vi "Example_OE1201 Control.vi"() -> ()   [LabVIEW 2011]
panel:
  in  "Sample count":u32
  out "Gain Overlaod":bool
  in  "Remote Mode":u16(ring) items=["USB", "RS232"]
  out "Freq":dbl
  out "xita":dbl
  out "R":dbl
  out "Input Overlaod":bool
  out "PLL Lock":bool
  out "Error":string
  out "Serial Versions":string
  in  "Table":T1(tab) caption="选项卡控件"
  in  "OE1201_Configure Input Filter":T2 {"Input Notch Filter" items=["None", "50Hz", "100Hz", "Both"]; "Input Coupling" items=["AC", "DC"]; "Input Shield Grounding" items=["Float", "Ground"]; "Input Source" items=["A", "B", "I-1M", "I-100M"]}
  in  "OE1201_Configure Ref Phase":T3={"Internal Frequency(Hz)"=1000.0, "External Ref Trigger"=0, "Reference Source"=0, "Phase  (degree)"=0.0} {"Phase  (degree)" format="%#.2g"; "Reference Source" items=["External", "Internal"]; "External Ref Trigger" items=["TTL Rising Edge", "Sine Zero Crossing"]; "Internal Frequency(Hz)" min=0.001 max=120000.0 format="%#_10g"}
  in  "OE1201_Configure Sens and Filter":T4={"Dynamic Reserve"=1, "Sensitivity "=24, "Time Constant "=9, "Low Pass Filter Slope "=1, "Enable Sync Filter "=0} {"Enable Sync Filter" items=["OFF", "ON"]; "Low Pass Filter Slope" items=["6 dB/oct", "12 dB/oct", "18 db/oct", "24 dB/oct"]; "Time Constant" items=["10 us", "30 us", "100 us", "300 us", "1 ms", "3 ms", "10 ms", "30 ms", "100 ms", "300 ms", "1 s", "3 s", "10 s", "30 s", "100 s", "300 s", "1 ks", "3 ks"]; "Sensitivity" items=["2 nV/fA", "5 nV/fA", "10 nV/fA", "20 nV/fA", "50 nV/fA", "100 nV/fA", "200 nV/fA", "500 nV/fA", "1 uV/pA", "2 uV/pA", "5 uV/pA", "10 uV/pA", "20 uV/pA", "50 uV/pA", "100 uV/pA", "200 uV/pA", "500 uV/pA", "1 mV/nA", "2 mV/nA", "5 mV/nA", "10 mV/nA", "20 mV/nA", "50 mV/nA", "100 mV/nA", "200 mV/nA", "500 mV/nA", "1 V/uA"]; "Dynamic Reserve" items=["High Reserve", "Normal", "Low Noise"]}
  in  "OE1201_Configure Channel Out":T5={"CH 1"=0, "CH 2"=0, "CH2 Offset(%)"=0.0, "CH1 Offset(%)"=0.0, "CH2 Expand"=1, "CH1 Expand"=1} {"CH1 Expand" min=1 max=256; "CH2 Expand" min=1 max=256; "CH1 Offset(%)" min=-100.0 max=100.0 format="%#.2g"; "CH2 Offset(%)" min=-100.0 max=100.0 format="%#.2g"; "CH 2" items=["R"=3, "X"=1, "Y"=2, "θ"=4]; "CH 1" items=["R"=3, "X"=1, "Y"=2, "θ"=4]}
  in  "OE1201_Configure Sine Out":cluster{"Sine Output Amplitude (V)":dbl}={"Sine Output Amplitude (V)"=0.1} {"Sine Output Amplitude (V)" min=0.1 max=1.0 format="%.3f"}
  in  "OE1201_Configure Harmonic":cluster{"Harmonic":u16}={"Harmonic"=1} {"Harmonic" min=1 max=32767}
  in  "Sample Rate":dbl=0.1 min=0.1 max=100.0
  in  "Save Button":bool
  in  "file path":path
  out "Status":string
  in  "Connect":bool
  in  "VISA resource name":refnum<visa-resource-name>
  in  "Baud Rate (921600)":u32=921600
  # "Tel          :   +86-020-84133345\nWebsite  :   www.ssi-instrument.com\nE-mail     :   support@si-instrument.com"
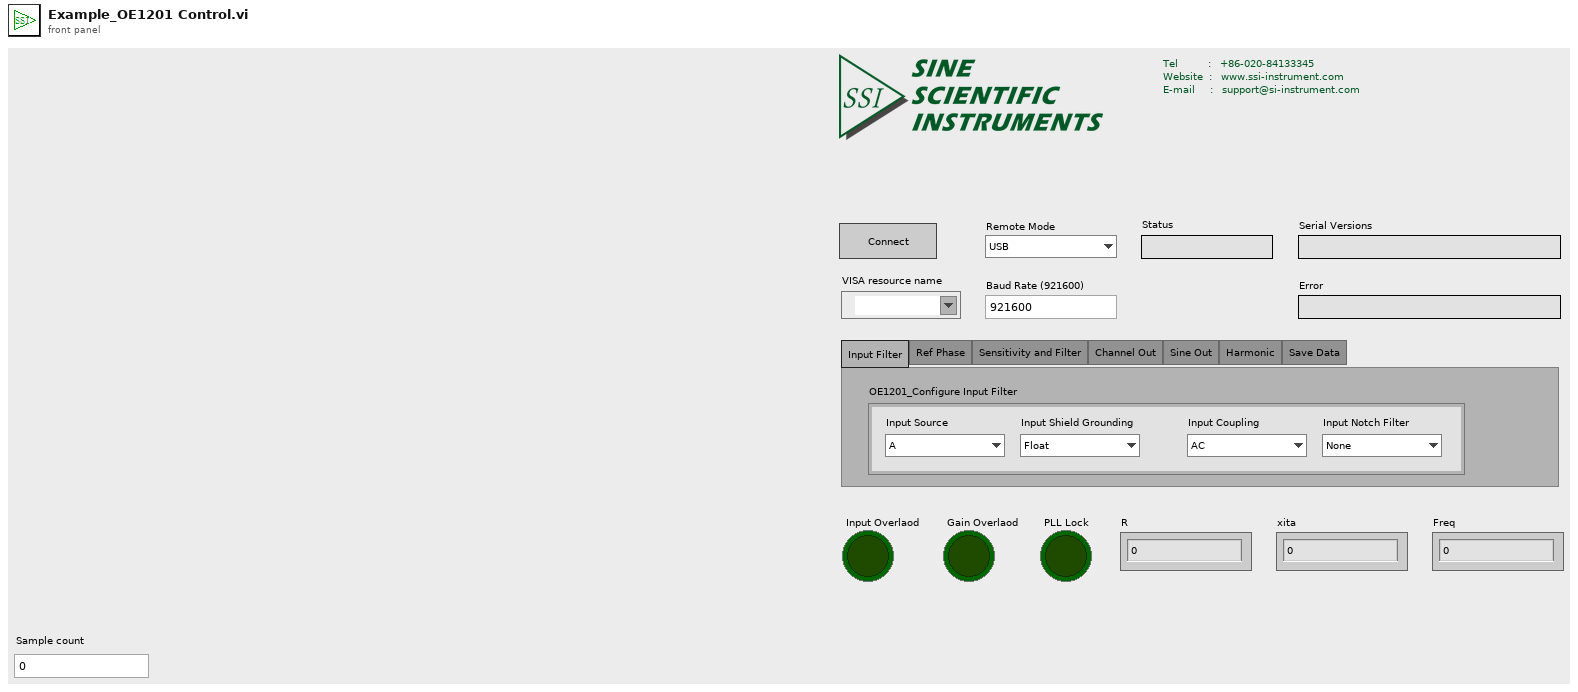
[diagram p1: front panel]
types:
  T1 = enum32{"Input Filter", "Ref Phase", "Sensitivity and Filter", "Channel Out", "Sine Out", "Harmonic", "Save Data"}
  T2 = cluster{"Input Source":u16, "Input Shield Grounding ":u16, "Input Coupling ":u16, "Input Notch Filter ":u16}
  T3 = cluster{"Internal Frequency(Hz)":dbl, "External Ref Trigger":u16, "Reference Source":u16, "Phase  (degree)":dbl}
  T4 = cluster{"Dynamic Reserve":u16, "Sensitivity ":u16, "Time Constant ":u8, "Low Pass Filter Slope ":u8, "Enable Sync Filter ":u16}
  T5 = cluster{"CH 1":i8, "CH 2":i8, "CH2 Offset(%)":dbl, "CH1 Offset(%)":dbl, "CH2 Expand":u16, "CH1 Expand":u16}
  T6 = enum16{"OE1022", "OE1022D", "OE1201", "OE2031&OE2041", "OE1311&OE1351"}
  T7 = cluster{"Input Overlaod":bool, "Gain Overlaod":bool, "PLL Lock(1: External Lock)":bool}
  T8 = cluster{"R":dbl, "X":dbl, "Y":dbl, "θ":dbl, "Freq":dbl}
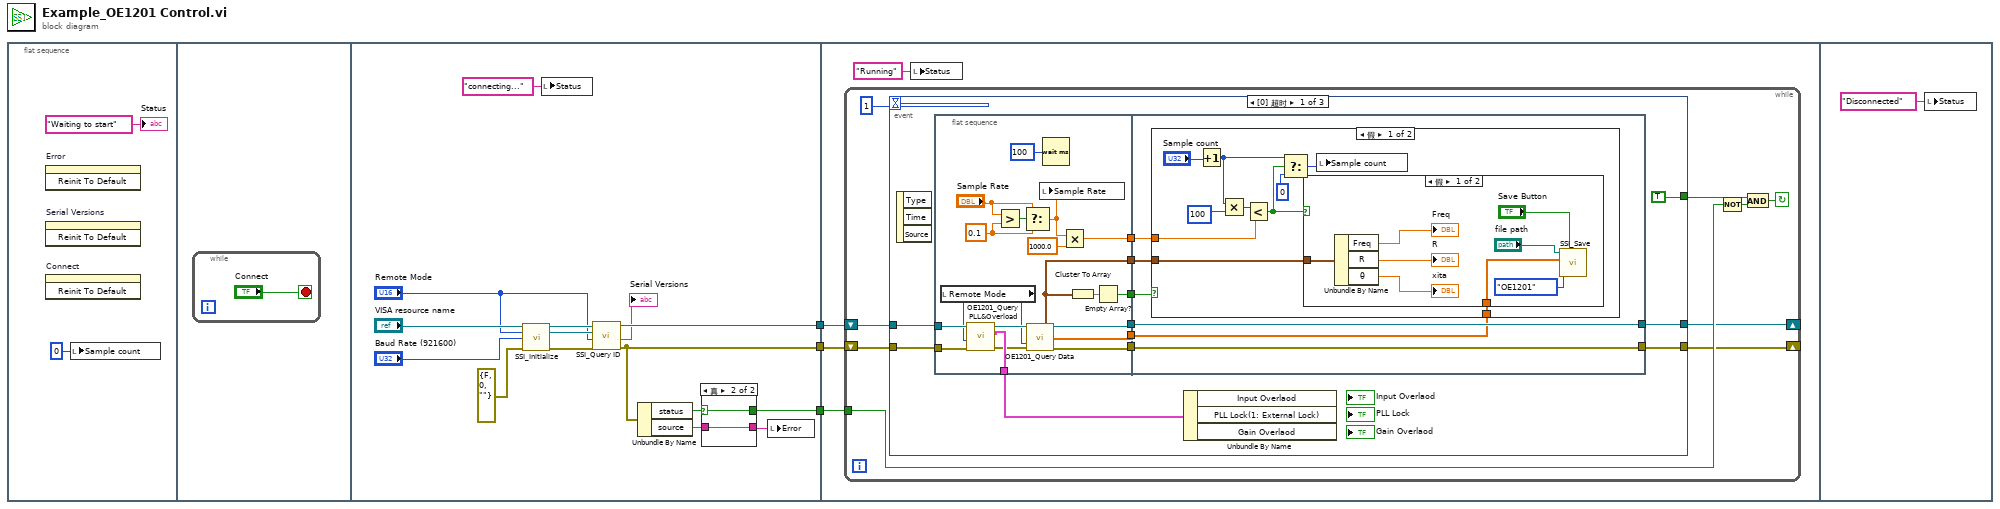
[diagram p0: block diagram]
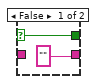
[diagram p2: hidden frame]
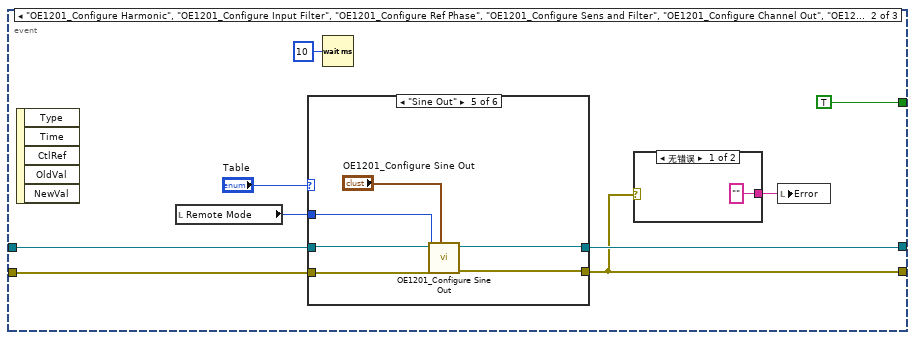
[diagram p5: hidden frame]
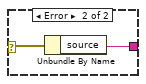
[diagram p6: hidden frame]
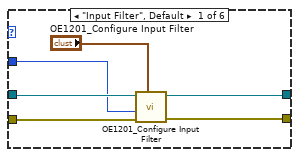
[diagram p7: hidden frame]
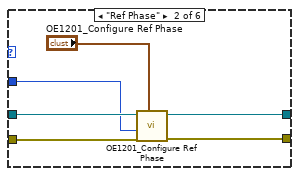
[diagram p8: hidden frame]
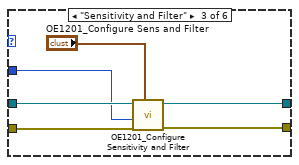
[diagram p9: hidden frame]
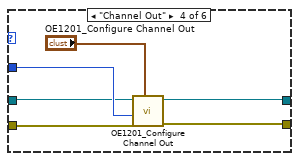
[diagram p10: hidden frame]
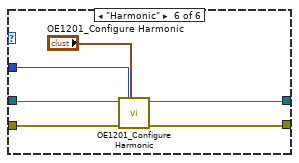
[diagram p11: hidden frame]
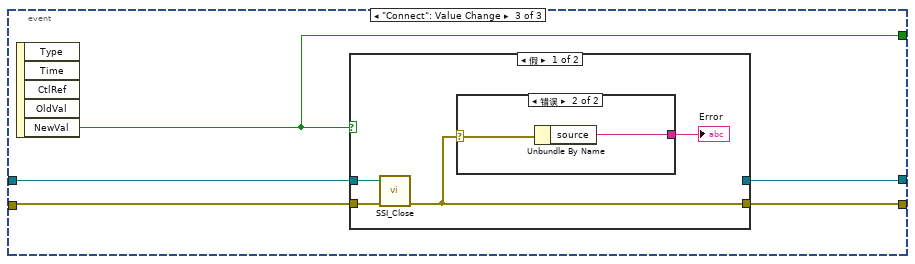
[diagram p12: hidden frame]
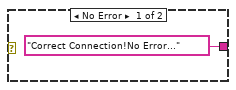
[diagram p13: hidden frame]
diagram:
  n1 = flat-sequence {
    tunnel: [w15] -> w3
    tunnel: [w12] -> w2
    tunnel: [w10] -> w1
    tunnel: w3 -> [w28]
    tunnel: w2 -> [w27]
    tunnel: w1 -> [w26]
    frame #0 {
      n2 = invoke on="Error" class="Str" method="Reinit To Default"() -> ()  [unwired: 3 in, 3 out]
      n3 = invoke on="Serial Versions" class="Str" method="Reinit To Default"() -> ()  [unwired: 3 in, 3 out]
      n4 = invoke on="Connect" class="Bool (严格)" method="Reinit To Default"() -> ()  [unwired: 3 in, 3 out]
      n5 = local write "Sample count"(u32 0 ("Sample count")) -> ()
      "Status" <- "Waiting to start" ("status")
    }
    frame #1 {
      n6 = while {
        stop <- "Connect" stop-if-true
      }
    }
    frame #2 {
      n7 = call "SSI_Initialize.vi"("VISA resource name"="VISA resource name", "Remote Mode"="Remote Mode", "baud rate (921600)"="Baud Rate (921600)", "error in (no error)"=errorcluster {"status"=FALSE, "code"=0, "source"=""}) -> ("VISA resource name out"=w19:refnum<visa-resource-name>, "connection ID(Ethernet)"=w18:refnum<k5>, "error out"=w17:errorcluster)  [unwired: 9 in]
      n8 = local write "Status"("connecting..." ("status")) -> ()
      n9 = call "SSI_Query ID.vi"("Error in (no error)"=w17, "Remote Mode"="Remote Mode", "Connection ID in"=w18, "VISA resource name"=w19) -> ("Error out"=w12:errorcluster, "Read Buffer"=→"Serial Versions":string, "VISA resource  out"=w15:refnum<visa-resource-name>)  [unwired: 4 in, 1 out]
      n10 = Unbundle By Name(w12) -> ("status"=w11:bool, "source"=w9:string)
      n11 = case shown="真" w11 {
        selector: w11 -> [w23 w25]
        tunnel: [w23 w25] -> w10
        tunnel: ["" w24] -> w8
        tunnel: w9 -> [_ w24]
        frame False {
        }
        frame True {
        }
      }
      n12 = local write "Error"(w8) -> ()
    }
    frame #3 {
      n13 = while {
        tunnel: w26 -> [w34]
        shift-right: [w31] -> _
        shift-left: w28 -> [w32]
        shift-right: [w30] -> _
        shift-left: w27 -> [w33]
        stop <- w35 continue-if-true
        n14 = event shown="[0] 超时" {
          selector: _ -> [_ _ _]
          dyn-events: _ -> [_ _ _]
          timeout: 1 -> [_ _ _]
          tunnel: [TRUE ("Stop") TRUE ("Stop") w142] -> w36
          tunnel: [w45 w97 w144] -> w30
          tunnel: [w46 w99 w143] -> w31
          tunnel: w32 -> [w47 w101 w146]
          tunnel: w33 -> [w48 w100 w145]
          event Timeout {
            n15 = event-data() -> ()  [unwired: 1 in, 3 out]
            n16 = flat-sequence {
              tunnel: [w56] -> w44
              tunnel: [w57] -> w43
              tunnel: [w64] -> w42
              tunnel: [w63] -> w41
              tunnel: [w52] -> w40
              tunnel: [w53] -> w39
              tunnel: [w55] -> w49
              tunnel: w48 -> [w59]
              tunnel: w47 -> [w60]
              tunnel: w44 -> [w74]
              tunnel: w43 -> [w75]
              tunnel: [w75] -> w46
              tunnel: [w74] -> w45
              tunnel: w42 -> [w71]
              tunnel: w41 -> [w70]
              tunnel: w40 -> [w72]
              tunnel: w39 -> [w73]
              frame #0 {
                w67 = 0.1 ("y")
                n17 = local read "Remote Mode"() -> (w51:u16)
                n18 = call "OE1201_Query PLL&Overload.vi"("Error in (no error)"=w59, "Remote Mode"=w51, "VISA resource name"=w60) -> ("Error out"=w54:errorcluster, "OE1201_Query PLL&Overload"=w55:T7, "VISA resource  out"=w58:refnum<visa-resource-name>)  [unwired: 5 in, 1 out]
                n19 = Greater?(x="Sample Rate", y=w67) -> (0:w66:bool)
                n20 = Select(t="Sample Rate", s=w66, f=w67) -> (s? t:f=w65:dbl)
                n21 = call "OE1201_Query Data.vi"("VISA resource name"=w58, "Remote Mode"=w51, "Error in (no error)"=w54) -> ("VISA resource  out"=w57:refnum<visa-resource-name>, "Parameter Values"=w52:T8, "Data Array"=w53:dbl[], "Error out"=w56:errorcluster)  [unwired: 8 in, 1 out]
                n22 = local write "Sample Rate"(w65) -> ()
                n23 = Wait (ms)(milliseconds to wait=u32 100 ("等待时间（毫秒）")) -> ()  [unwired: 1 out]
                n24 = Multiply(x=w65, y=1000.0) -> (x*y=w63:dbl)
                n25 = Cluster To Array(cluster=w52) -> (array=w69:dbl[])
                n26 = Empty Array?(array=w69) -> (empty?=w64:bool)
              }
              frame #1 {
                n27 = case shown="假" w71 {
                  tunnel: w73 -> [w85 _]
                  tunnel: w72 -> [w84 _]
                  tunnel: w70 -> [w81 _]
                  frame False {
                    n28 = Increment(x="Sample count") -> (x+1=w77:u32)
                    n29 = Multiply(x=w77, y=u32 100) -> (x*y=w82:u32)
                    n30 = Less?(x=w82, y=w81) -> (x < y?=w79:bool)
                    n31 = Select(t=w77, s=w79, f=0) -> (s? t:f=w78:u32)
                    n32 = case shown="假" w79 {
                      tunnel: w84 -> [w93 _]
                      tunnel: w85 -> [w92 _]
                      frame False {
                        n33 = Unbundle By Name(w93) -> ("Freq"=→"Freq":dbl, "R"=→"R":dbl, "θ"=→"xita":dbl)
                        n34 = call "SSI_Save.vi"("file path (dialog if empty)"="file path", "1D data"=w92, "Instrument Mode"=T6."OE1201", "Save Button"="Save Button") -> ()  [unwired: 7 in]
                      }
                      frame True {
                      }
                    }
                    n35 = local write "Sample count"(w78) -> ()
                  }
                  frame True {
                  }
                }
              }
            }
            n36 = Unbundle By Name(w49) -> ()  [unwired: 3 out]
          }
          event "OE1201_Configure Harmonic", "OE1201_Configure Input Filter", "OE1201_Configure Ref Phase", "OE1201_Configure Sens and Filter", "OE1201_Configure Channel Out", "OE1201_Configure Sine Out": Value Change {
            n37 = event-data() -> ()  [unwired: 1 in, 5 out]
            n38 = local read "Remote Mode"() -> (w95:u16)
            n39 = case shown="\"Sine Out\"" "Table" {
              tunnel: w101 -> [w110 w117 w123 w127 w132 w139]
              tunnel: w100 -> [w111 w116 w122 w129 w135 w141]
              tunnel: [w108 w115 w120 w125 w133 w138] -> w99
              tunnel: [w109 w114 w121 w126 w134 w137] -> w97
              tunnel: w95 -> [w107 w113 w119 w128 w131 w140]
              frame "Input Filter", Default {
                n40 = call "OE1201_Configure Input Filter.vi"("OE1201_Configure Input Filter"="OE1201_Configure Input Filter", "Error in (no error)"=w111, "Remote Mode"=w107, "VISA resource name"=w110) -> ("Error out"=w109:errorcluster, "VISA resource  out"=w108:refnum<visa-resource-name>)  [unwired: 5 in, 1 out]
              }
              frame "Ref Phase" {
                n41 = call "OE1201_Configure Ref Phase.vi"("OE1201_Configure Ref Phase"="OE1201_Configure Ref Phase", "Error in (no error)"=w116, "Remote Mode"=w113, "VISA resource name"=w117) -> ("Error out"=w114:errorcluster, "VISA resource  out"=w115:refnum<visa-resource-name>)  [unwired: 5 in, 1 out]
              }
              frame "Sensitivity and Filter" {
                n42 = call "OE1201_Configure Sensitivity and Filter.vi"("OE1201_Configure Sens and Filter"="OE1201_Configure Sens and Filter", "Error in (no error)"=w122, "Remote Mode"=w119, "VISA resource name"=w123) -> ("Error out"=w121:errorcluster, "VISA resource  out"=w120:refnum<visa-resource-name>)  [unwired: 5 in, 1 out]
              }
              frame "Channel Out" {
                n43 = call "OE1201_Configure Channel Out.vi"("OE1201_Configure Channel Out"="OE1201_Configure Channel Out", "Error in (no error)"=w129, "Remote Mode"=w128, "VISA resource name"=w127) -> ("Error out"=w126:errorcluster, "VISA resource  out"=w125:refnum<visa-resource-name>)  [unwired: 5 in, 1 out]
              }
              frame "Sine Out" {
                n44 = call "OE1201_Configure Sine Out.vi"("OE1201_Configure Sine Out"="OE1201_Configure Sine Out", "Error in (no error)"=w135, "Remote Mode"=w131, "VISA resource name"=w132) -> ("Error out"=w134:errorcluster, "VISA resource  out"=w133:refnum<visa-resource-name>)  [unwired: 5 in, 1 out]
              }
              frame "Harmonic" {
                n45 = call "OE1201_Configure Harmonic.vi"("OE1201_Configure Harmonic"="OE1201_Configure Harmonic", "Error in (no error)"=w141, "Remote Mode"=w140, "VISA resource name"=w139) -> ("Error out"=w137:errorcluster, "VISA resource  out"=w138:refnum<visa-resource-name>)  [unwired: 5 in, 1 out]
              }
            }
            n46 = Wait (ms)(milliseconds to wait=u32 10 ("等待时间（毫秒）")) -> ()  [unwired: 1 out]
            n47 = case shown="无错误" w97 {
              selector: w97 -> [_ w105]
              tunnel: ["" ("source") w104] -> w96
              frame No Error {
              }
              frame Error {
                n48 = Unbundle By Name(w105) -> ("source"=w104:string)
              }
            }
            n49 = local write "Error"(w96) -> ()
          }
          event "Connect": Value Change {
            n50 = event-data() -> ("NewVal"=w142:bool)  [unwired: 1 in, 4 out]
            n51 = case shown="假" w142 {
              tunnel: w146 -> [w150 w155]
              tunnel: w145 -> [w149 w154]
              tunnel: [w148 w154] -> w144
              tunnel: [_ w155] -> w143
              frame False {
                n52 = call "SSI_Close.vi"("Error in (no error)"=w149, "VISA resource name"=w150) -> ("Error out"=w148:errorcluster)  [unwired: 5 in]
                n53 = case shown="错误" w148 {
                  selector: w148 -> [_ w153]
                  tunnel: ["Correct Connection!No Error..." ("source") w152] -> w147
                  frame No Error {
                  }
                  frame Error {
                    n54 = Unbundle By Name(w153) -> ("source"=w152:string)
                  }
                }
                "Error" <- w147
              }
              frame True {
              }
            }
          }
        }
        n55 = Not(x=w34) -> (.not. x?=w37:bool)
        n56 = And(x=w36, y=w37) -> (x .and. y?=w35:bool)
      }
      n57 = local write "Status"("Running" ("status")) -> ()
    }
    frame #4 {
      n58 = local write "Status"("Disconnected" ("status")) -> ()
    }
  }
